vi "AlliGator Apply Calibration Phasor(s) v2.vi"(6 "Phasor Frequency":dbl[unit], 7 "Phasor Graph Ref":refnum<vi>, 8 "Error In":errorcluster, 9 "Plot Index (-1: last)":i32, 10 "Phasor Graph Ctrl Refnums":T1, 11 "AlliGator IV DVR":refnum<data-value>) -> (0 "Error Out":errorcluster, 1 "Apparent Phase Lifetime":dbl[unit], 2 "Calibrated Phasor":T2, 3 "AlliGator IV DVR":refnum<data-value>, 4 "Message":string)   [LabVIEW 2021, in "AlliGator Phasor Calibration.lvlib"]
doc: "Calibrates single, selected or all plots.\nUpdates the Phasor Graph and internal variables."
uses:
  AlliGator Phasor Calibration.lvlib
  Phasor/Phasor (g, s).ctl
  Internal Variables/AlliGator Internal Variables v2.ctl
  <vilib>/vision/Image Controls.llb/IMAQ Image.ctl
  Internal Variables/AlliGator Gate Image Set.ctl
  Files/AlliGator FLI Dataset Type.ctl
  Files/AlliGator Data Series Type.ctl
  Dual-Channel Datasets/AlliGator Dataset Channel.ctl
  Settings/AlliGator Gate Arithmetic.ctl
  Source Image/AlliGator Displayed Image.ctl
  Image/Named ROI Description.ctl
  Phasor Graph/AlliGator Decay Metadata v3.ctl
  Decay Analysis/Decay Preprocessing/AlliGator Decay Background Subtraction Info.ctl
  Decay Analysis/Decay Preprocessing/AlliGator Baseline Subtraction Method.ctl
  Graphs/XY Graph/XY Graph Plot Shift Parameters.ctl
  Graphs/XY Graph/XY Graph Plot Shift Method.ctl
  Decay Analysis/Decay Preprocessing/AlliGator Decay Extrapolation Parameters.ctl
  Phasor/Calibration Phasor (m, phi).ctl
  Phasor/Phasor Reference Series.ctl
  Phasor/Phasor Calibration Map v2.ctl
  Phasor Graph/AlliGator Raw Phasor Plot Data v5.ctl
  Phasor/Phasor Standard Deviation Options.ctl
  Phasor Plot/AlliGator Phasor Multi-Harmonic Data.ctl
  Phasor/Phasor Harmonic Data.ctl
  Decay Fit Parameter Map/AlliGator Decay Fit Options & Parameters v4.ctl
  Fits/IRF(X)PSED/Decay Fit Options v4.ctl
  Fits/Decay Convolution/Decay Model.ctl
  Fits/Residual Type.ctl
  Fits/IRF(X)PSED/Fit Weights Type v2.ctl
  Fits/Non-linear Fitting Method v2.ctl
  Fits/Fit Calculation Method.ctl
  Fits/Non-linear Fitting Algorithm.ctl
  Decay Analysis/Decay Fit/AlliGator Decay Fit Parameter Constraints 2.ctl
  Fits/IRF(X)PSED/Decay Fit Parameters In List.ctl
  Fits/IRF(X)PSED/MLE Baseline Offset Type.ctl
  Decay Analysis/Decay Preprocessing/AlliGator Decay Preprocessing Parameters.ctl
  Fits/IRF(X)PSED/Decay Fit Parameters & Derived Quantities List v2.ctl
  Fits/IRF(X)PSED/Decay Fit Result Constraint.ctl
  Decay Fit Parameter Map/AlliGator Parameter Maps Data.ctl
  GUI/AlliGator Phasor Graph Ctrl Refnums.ctl
  Phasor/Phasor Calibration Type.ctl
  Arrays/Arrays.lvlib
  Strings/Strings.lvlib
  Phasor/Phasor.lvlib
  Time/Time.lvlib
  Internal Variables/AlliGator Internal Variables.lvlib
  Image/Image.lvlib
  Files/AlliGator Files.lvlib
  Phasor Graph/AlliGator Phasor Graph.lvlib
  Decay Analysis/Decay Preprocessing/AlliGator Decay Preprocessing.lvlib
  Graphs/XY Graph/XY Graph Add-Ons.lvlib
  Phasor Plot/AlliGator Phasor Plot.lvlib
  Source Image/AlliGator Source Image.lvlib
  Fits/Fits.lvlib
  Decay Analysis/Decay Fit/AlliGator Decay Fit.lvlib
  GUI/AlliGator GUI.lvlib
  Settings/AlliGator Settings.lvlib
  Dual-Channel Datasets/AlliGator Dual-Channel Datasets.lvlib
  Decay Fit Parameter Map/AlliGator Decay Fit Parameter Map.lvlib
panel:
  out "# Plots":i32
  # "see the AlliGator License on the block diagram (Ctrl+E or Window:Show Block Diagram)"
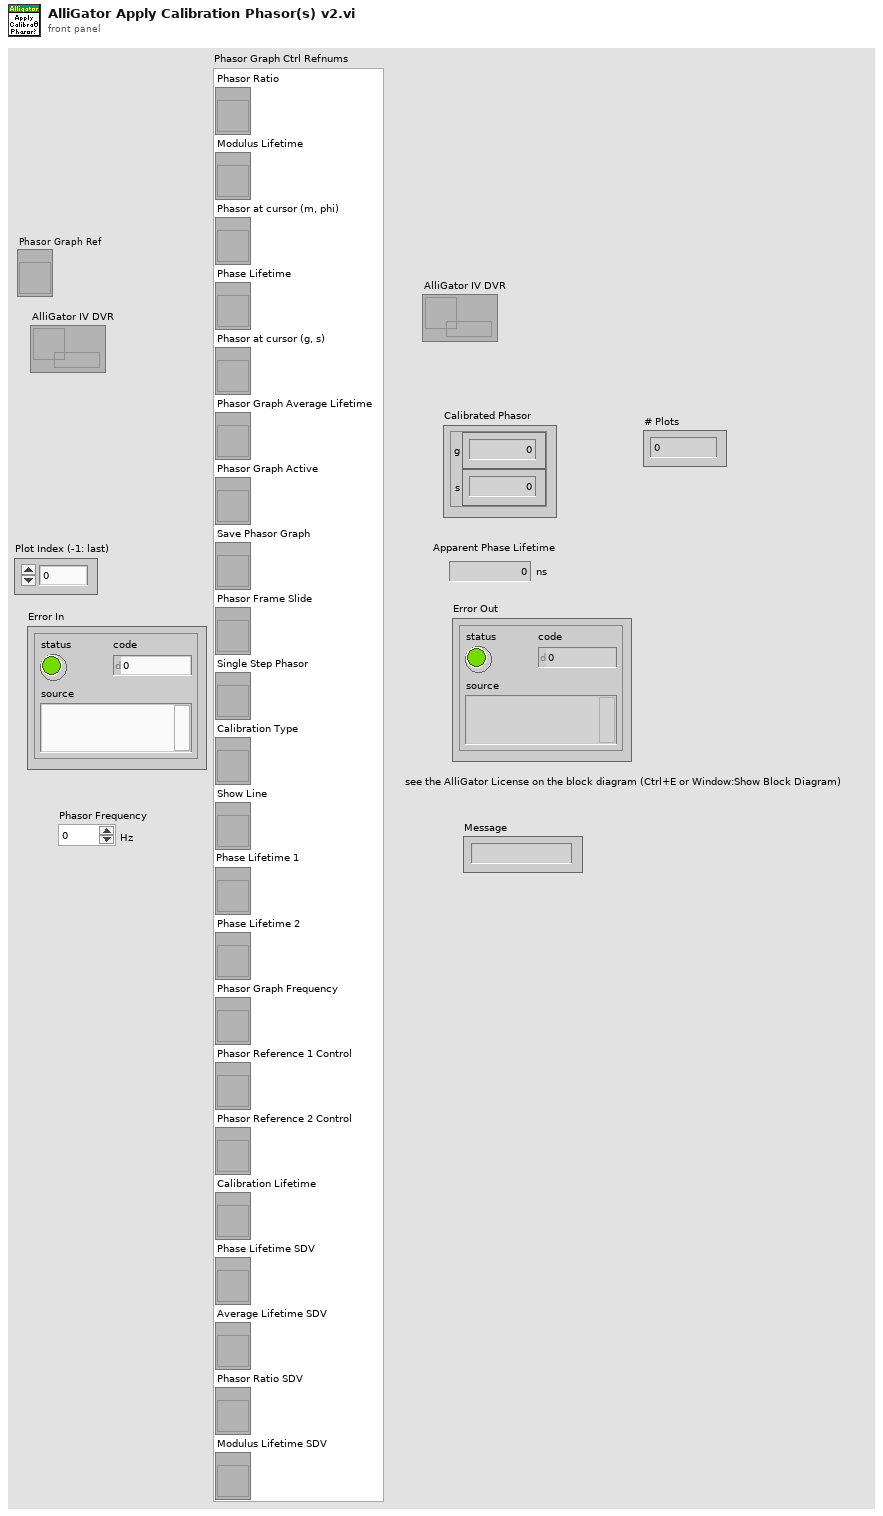
[diagram p1: front panel]
types:
  T1 = typedef "AlliGator GUI.lvlib/AlliGator Phasor Graph Ctrl Refnums.ctl" = cluster{"Phasor Ratio":refnum<vi>, "Modulus Lifetime":refnum<vi>, "Phasor at cursor (m, phi)":refnum<vi>, "Phase Lifetime":refnum<vi>, "Phasor at cursor (g, s)":refnum<vi>, "Phasor Graph Average Lifetime":refnum<vi>, "Phasor Graph Active":refnum<vi>, "Save Phasor Graph":refnum<vi>, "Phasor Frame Slide":refnum<vi>, "Single Step Phasor":refnum<vi>, "Calibration Type":refnum<vi>, "Show Line":refnum<vi>, "Phase Lifetime 1":refnum<vi>, "Phase Lifetime 2":refnum<vi>, "Phasor Graph Frequency":refnum<vi>, "Phasor Reference 1 Control":refnum<vi>, "Phasor Reference 2 Control":refnum<vi>, "Calibration Lifetime":refnum<vi>, "Phase Lifetime SDV":refnum<vi>, "Average Lifetime SDV":refnum<vi>, "Phasor Ratio SDV":refnum<vi>, "Modulus Lifetime SDV":refnum<vi>}
  T2 = typedef "Phasor.lvlib/Phasor (g, s).ctl" = cluster{"g":dbl, "s":dbl}
  T3 = typedef "AlliGator Internal Variables.lvlib/AlliGator Internal Variables v2.ctl" = cluster{"----------------------------- Images -----------------------------":u8, "Displayed Image":T4, "White Light Image":T4, "Mask Image":T4, "ROI Mask Image":T4, "Current Dataset Images 1":T5, "Background Dataset Images 1":T5, "Current Dataset Images 2":T5, "Background Dataset Images 2":T5, "Current Dataset Arithmetic Images":T5, "Accumulated Dataset Images 1":T5, "Accumulated Dataset Images 2":T5, "Accumulated Dataset Arithmetic Images":T5, "----------------------------- File Paths -----------------------------":u8, "Phasor Plot Image":T4, "Decay Fit Parameter Map Image":T4, "Parameter Map Image":T4, "Single Data Point Path":path, "White Light Image Path":path, "Mask Image Path":path, "Time-Series Folder":path, "[Time-Series Paths]":path[], "----------------------------- FLI Dataset -----------------------------":u8, "Current Dataset":i32, "Single Dataset Type":T6, "Current Folder":string, "AlliGator Data Series Type":T7, "# Datasets":i32, "Dual-Channel Dataset":bool, "Selected Channel Name":string, "Dataset Channel":T8, "Channel Arithmetic":T9, "Dual-Channel Background Dataset":bool, "Background Channel":T8, "Dual-Channel Accumulated Dataset":bool, "Start Time":dbl, "[Time-Series Timestamps]":dbl[], "[Intensity Corrections]":dbl[], "Time Series Script":bool, "Type of Displayed Image":T10, "Gate Image Slide":u16, "# Gates":i32, "ROIs":T11[], "----------------------------- Decays -----------------------------":u8, "ROI Decay":cluster{"t Array":dbl[], "I Array":dbl[]}, "Valid Decay":bool, "Decay  Metadata":T13, "Reference Decay Plot Name":string, "Reference Decay":cluster{"t Array":dbl[], "I Array":dbl[]}, "Decay Shift Plot":cluster{"Time Stamps":dbl[], "Decay Shifts":dbl[]}, "[Decays Max Values]":sgl[], "[Decays Min Values]":sgl[], "----------------------------- Calibration -----------------------------":u8, "Calibration Phasor":T19, "Calibration Phasor Series":T20, "Phasor Calibration Map":T21, "Calibration Map MD5 Digest":string, "----------------------------- Phasor Graph -----------------------------":u8, "Last Raw Phasor":T2, "Last Calibrated Phasor":T2, "Last Calibrated Phasor SDV":T2, "Phasor Graph:Phasor Plot":cluster{"g Array":dbl[], "s Array":dbl[]}, "Phasor Graph:Phasor SDV Plot":cluster{"g Array":dbl[], "s Array":dbl[]}, "[Phasor Graph:Raw Phasor Plots]":T22[], "Phasor Plot locked to Ref 1":i32, "[Phasor Plot(s) locked to Ref 1]":i32[], "[Phasor Plot(s) locked to Ref 2]":i32[], "[Pixel Phasors]":T2[], "----------------------------- Phasor Plot -----------------------------":u8, "[[Sum Image]]":dbl[][], "[[CSG Phasors]]":csg[][], "[[Valid Pixel?]]":bool[][], "[[Phasor Ratios]]":dbl[][], "[[Average Lifetimes]]":dbl[][], "Amplitude Weighted Average Lifetime":bool, "I/m/phi Dataset":cluster{"I/m/phi Dataset?":bool, "Base Frequency":dbl[unit], "Harmonic Orders":u8[]}, "Multi Phasor Plot Data":T24, "----------------------------- Decay Fit Parameter Map -----------------------------":u8, "Decay Fit Options & Parameters":T26, "Fit Options: Decay Preprocessing Parameters":T37, "Fit Options: Reference Decay":cluster{"t Array":dbl[], "I Array":dbl[]}, "Is Full Image Parameters Map":bool, "Is Single-Pixels Parameters Map":bool, "NLSF Parameters Map X Resolution":i32, "NLSF Parameters Map Y Resolution":i32, "[Single Decay Fit Parameters]":dbl[], "Fit Model":T28, "[[Multiple Decays Fit Parameters]]":dbl[][], "[[Multiple Decays Fit Parameter SDVs]]":dbl[][], "[[IRFs]]":dbl[][], "[ROI Descriptors]":T12[], "IRF Array Time Axis":dbl[], "Decay Array Time Axis":dbl[], "[Decay Fit Parameter Names]":T38[], "[Decay Sum]":dbl[], "Array of Decay Fit Result Constraints":T39[], "Selected ROIs Array":bool[], "----------------------------- Parameter Maps -----------------------------":u8, "[Map Set Names]":string[], "[Parameter Maps]":T40[], "[[User-defined Quantities]]":dbl[][], "User-defined Quantity":string}
  T4 = typedef "IMAQ Image.ctl" = refnum<image>
  T5 = typedef "AlliGator Internal Variables.lvlib/AlliGator Gate Image Set.ctl" = cluster{"SGL Image Max":T4, "SGL Image Sum":T4, "SGL Gate Images":T4[], "SGL Image Min":T4}
  T6 = typedef "AlliGator Files.lvlib/AlliGator FLI Dataset Type.ctl" = enum16{"HDF5 FLI Dataset", "Gate Image Folder", ".sdt FLI Dataset (Becker & Hickl)", ".ptu FLI Dataset (PicoQuant)", "SS1 FLI Dataset", "SS2 FLI Dataset", "I/m/phi Dataset", ".bin FLI Dataset (PicoQuant Binned)", ".bin FLI Dataset (Piccolo Binned)", ".mat FLI Dataset"}
  T7 = typedef "AlliGator Files.lvlib/AlliGator Data Series Type.ctl" = enum16{"Not a Supported Series", "Gate Images Folder Series", "SwissSPAD 2 Dataset Series", "B&H FLI Dataset Series", "PicoQuant PTU FLI Dataset Series", "PicoQuant BIN FLI Dataset Series", "Piccolo hist BIN FLI Dataset Series", "HDF5 FLI Dataset Series"}
  T8 = typedef "AlliGator Dual-Channel Datasets.lvlib/AlliGator Dataset Channel.ctl" = enum16{"G2", "INT"}
  T9 = typedef "AlliGator Settings.lvlib/AlliGator Gate Arithmetic.ctl" = enum16{"None", "INT-G2", "G2/INT*<INT>", "(1 - G2/INT)*<INT>"}
  T10 = typedef "AlliGator Source Image.lvlib/AlliGator Displayed Image.ctl" = enum16{"Single Gate", "Sum of All Gates", "Max of All Gates", "Min of All Gates", "-", "White Ligth Image", "Mask Image"}
  T11 = typedef "Image.lvlib/Named ROI Description.ctl" = cluster{"ROI Descriptor":T12, "ROI Name":string, "Overlay Color":u32}
  T12 = typedef "ROI Descriptor" = cluster{"Global Rectangle":i32[], "Contours":cluster{"ID":enum32{"External", "Internal"}, "Type":u32, "Coordinates":i32[]}[]}
  T13 = typedef "AlliGator Phasor Graph.lvlib/AlliGator Decay Metadata v3.ctl" = cluster{"ROI Descriptor":T12, "ROI Center":cluster{"X":i32, "Y":i32}, "Decay Background Subtraction Info":T14, "Decay Reverted":bool, "Decay Smoothened":bool, "Decay Straightened":bool, "Fitted Tau (Decay Straightening)":dbl, "Decay Shift Parameters":T16, "Decay Shifted":bool, "Decay Extrapolated":bool, "Decay Extrapolation Parameters":T18, "Decay Normalized":bool, "Fold Decay":bool, "# Folds":u32}
  T14 = typedef "AlliGator Decay Preprocessing.lvlib/AlliGator Decay Background Subtraction Info.ctl" = cluster{"Laser Period":dbl[unit], "Gate Duration":dbl[unit], "Baseline Subtraction Method":T15, "Background Definition Range":cluster{"Min Gate":dbl[unit], "Max Gate":dbl[unit]}, "Total Intensity w/o Bkgd Subtraction":dbl, "Bkgd-subtracted Intensity (exp)":dbl, "# Data Points":i32, "Background/Gate":dbl, "Fitted Lifetime":dbl[unit], "Bkgd-subtracted Intensity (theo)":dbl}
  T15 = typedef "AlliGator Decay Preprocessing.lvlib/AlliGator Baseline Subtraction Method.ctl" = enum16{"Mean", "Min", "Square Gated Single-Exponential", "File", "Constant"}
  T16 = typedef "XY Graph Add-Ons.lvlib/XY Graph Plot Shift Parameters.ctl" = cluster{"Type":T17, "Shift":dbl[unit], "Threshold":dbl, "Rotate":bool}
  T17 = typedef "XY Graph Add-Ons.lvlib/XY Graph Plot Shift Method.ctl" = enum16{"Default", "CFD", "Threshold", "Cross-Correlation"}
  T18 = typedef "AlliGator Decay Preprocessing.lvlib/AlliGator Decay Extrapolation Parameters.ctl" = cluster{"Additional Points":u32, "Head Fraction":dbl, "Fitted Tau":dbl, "Use Periodicity":bool, "Use Cursors":bool, "Tail Fraction":dbl}
  T19 = typedef "Phasor.lvlib/Calibration Phasor (m, phi).ctl" = cluster{"m":dbl, "phi":dbl, "Phasor Frequency":dbl[unit], "Reference Lifetime":dbl[unit]}
  T20 = typedef "Phasor.lvlib/Phasor Reference Series.ctl" = cluster{"m Array":dbl[], "phi Array":dbl[], "Phasor Frequency":dbl[unit], "Calibration Lifetime":dbl[unit]}
  T21 = typedef "Phasor.lvlib/Phasor Calibration Map v2.ctl" = cluster{"Phasor Frequency":dbl[unit], "Calibration Lifetime":dbl[unit], "ROI Centers":cluster{"X":i32, "Y":i32}[], "ROI Descriptors":T12[], "Map Resolution X":i32, "Map Resolution Y":i32, "z Array":cdb[]}
  T22 = typedef "AlliGator Phasor Graph.lvlib/AlliGator Raw Phasor Plot Data v5.ctl" = cluster{"Phasor Plot Name":string, "Raw Phasor Plot":T2[], "Phasor Frequency":dbl[unit], "[Decay Metadata]":T13[], "Raw Phasor Plot SDV":T2[], "Phasor SDV Options":T23, "[Calibration Phasor]":T19[], "Intensity Array":dbl[]}
  T23 = typedef "Phasor.lvlib/Phasor Standard Deviation Options.ctl" = cluster{"Compute Estimated SDV":bool, "# Replicas":u32, "Use Estimated Average Phasor":bool}
  T24 = typedef "AlliGator Phasor Plot.lvlib/AlliGator Phasor Multi-Harmonic Data.ctl" = cluster{"Base Frequency":dbl[unit], "# Harmonics":u8, "Harmonic Orders":u8[], "Phasor Plot Settings Checksum":u64, "Phasor Harmonic Data Array":T25[]}
  T25 = typedef "Phasor.lvlib/Phasor Harmonic Data.ctl" = cluster{"Phasor Harmonic Name":string, "Phasor Plot Settings Checksum":u64, "Phasor Frequency":dbl[unit], "Base Frequency":dbl[unit], "Harmonic Order":u8, "Phasor Plot Parameters":string, "Phasor Array [[CSG]]":csg[][], "Dataset File Path":path}
  T26 = typedef "AlliGator Decay Fit Parameter Map.lvlib/AlliGator Decay Fit Options & Parameters v4.ctl" = cluster{"SYNC Period":dbl[unit], "Fit Options":T27, "Fit Parameter Constraints":T34[], "MLE Baseline Offset":dbl, "MLE Baseline Offset Type":T36}
  T27 = typedef "Fits.lvlib/Decay Fit Options v4.ctl" = cluster{"Show Fit Residuals":bool, "Fit Model":T28, "Residual Type":T29, "Max Decay Percentile":dbl, "Min Decay Percentile":dbl, "Show Full Decay":bool, "Weights":T30, "Fitting Method":T31, "Compute Parameter Uncertainties":bool, "Periodic Boundaries":bool, "Model Calculation":T32, "Period":dbl[unit], "Termination Criteria":cluster{"Max Iterations":i32, "Max Function Calls":i32, "Max Time":dbl[unit], "Function Tolerance":dbl, "Parameter Tolerance":dbl, "Gradient Tolerance":dbl, "Min Lambda":dbl, "Max Lambda":dbl, "Initial Tick Count":u32}, "Offset Resolution":dbl[unit], "Use Local IRF":bool, "Fitting Algorithm":T33, "Show Confidence Interval ":bool, "Confidence Level":dbl}
  T28 = typedef "Fits.lvlib/Decay Model.ctl" = enum16{"1-Exponential", "2-Exponentials"}
  T29 = typedef "Fits.lvlib/Residual Type.ctl" = enum16{"Standard", "Normalized", "Reduced"}
  T30 = typedef "Fits.lvlib/Fit Weights Type v2.ctl" = enum16{"Unweighted", "1/Variance (Neyman)", "1/Variance (Pearson)", "Best of All"}
  T31 = typedef "Fits.lvlib/Non-linear Fitting Method v2.ctl" = enum16{"Least Square", "Least Absolute Residual", "Bisquare", "MLE", "-", "Best of All"}
  T32 = typedef "Fits.lvlib/Fit Calculation Method.ctl" = enum16{"Simulation", "Convolution", "Integration"}
  T33 = typedef "Fits.lvlib/Non-linear Fitting Algorithm.ctl" = enum16{"Levenberg-Marquardt", "Trust-Region Dogleg"}
  T34 = typedef "AlliGator Decay Fit.lvlib/AlliGator Decay Fit Parameter Constraints 2.ctl" = cluster{"Fit Parameter":T35, "Min Value":dbl, "Max Value":dbl, "Global":bool, "Used":bool}
  T35 = typedef "Fits.lvlib/Decay Fit Parameters In List.ctl" = enum16{"Offset", "Baseline", "A_1", "tau_1", "A_2", "tau_2"}
  T36 = typedef "Fits.lvlib/MLE Baseline Offset Type.ctl" = enum32{"Absolute", "Percentage"}
  T37 = typedef "AlliGator Decay Preprocessing.lvlib/AlliGator Decay Preprocessing Parameters.ctl" = cluster{"Background Subtraction":bool, "Straighten Decay":bool, "Reverse Gates":bool, "1-Normalized Decay":bool, "Smoothen Decay":bool, "Smoothing Parameter":dbl, "Shift Decay":bool, "Decay Shift Parameters":T16, "Extrapolate Decay":bool, "Additional Points":u32, "Head Fraction":dbl, "Pixel-Normalize Decay":bool, "Use Periodicity":bool, "Use Cursors":bool, "Tail Fraction":dbl, "Use Decay Pre-Processing":bool, "Fold Decay":bool, "# Folds":u32, "[0-1]-Normalized Decay":bool}
  T38 = typedef "Fits.lvlib/Decay Fit Parameters & Derived Quantities List v2.ctl" = enum16{"Offset", "Baseline", "A_1", "tau_1", "A_2", "tau_2", "<tau>_a", "f1_a", "f2_a", "<tau>_i", "f1_i", "f2_i", "-", "R^2", "Chi^2"}
  T39 = typedef "Fits.lvlib/Decay Fit Result Constraint.ctl" = cluster{"Fit Parameter":enum16{"Offset", "Baseline", "A_1", "tau_1", "A_2", "tau_2", "<tau>_a", "f1_a", "f2_a", "<tau>_i", "f1_i", "f2_i", "-", "R^2", "Chi^2", "Max Relative Residual", "<Residual ACF>", "Residual ACF SDV", "tau_2/tau_1"}, "Min Value":dbl, "Max Value":dbl, "Use Constraint":bool}
  T40 = typedef "AlliGator Decay Fit Parameter Map.lvlib/AlliGator Parameter Maps Data.ctl" = cluster{"Map Set Name":string, "[Parameter Names]":string[], "[[Parameters]]":dbl[][], "[[Parameter SDVs]]":dbl[][], "Decay Array Time Axis":dbl[], "[[IRFs]]":dbl[][], "IRF Array Time Axis":dbl[], "X Resolution":i32, "Y Resolution":i32, "Intensity Array":dbl[]}
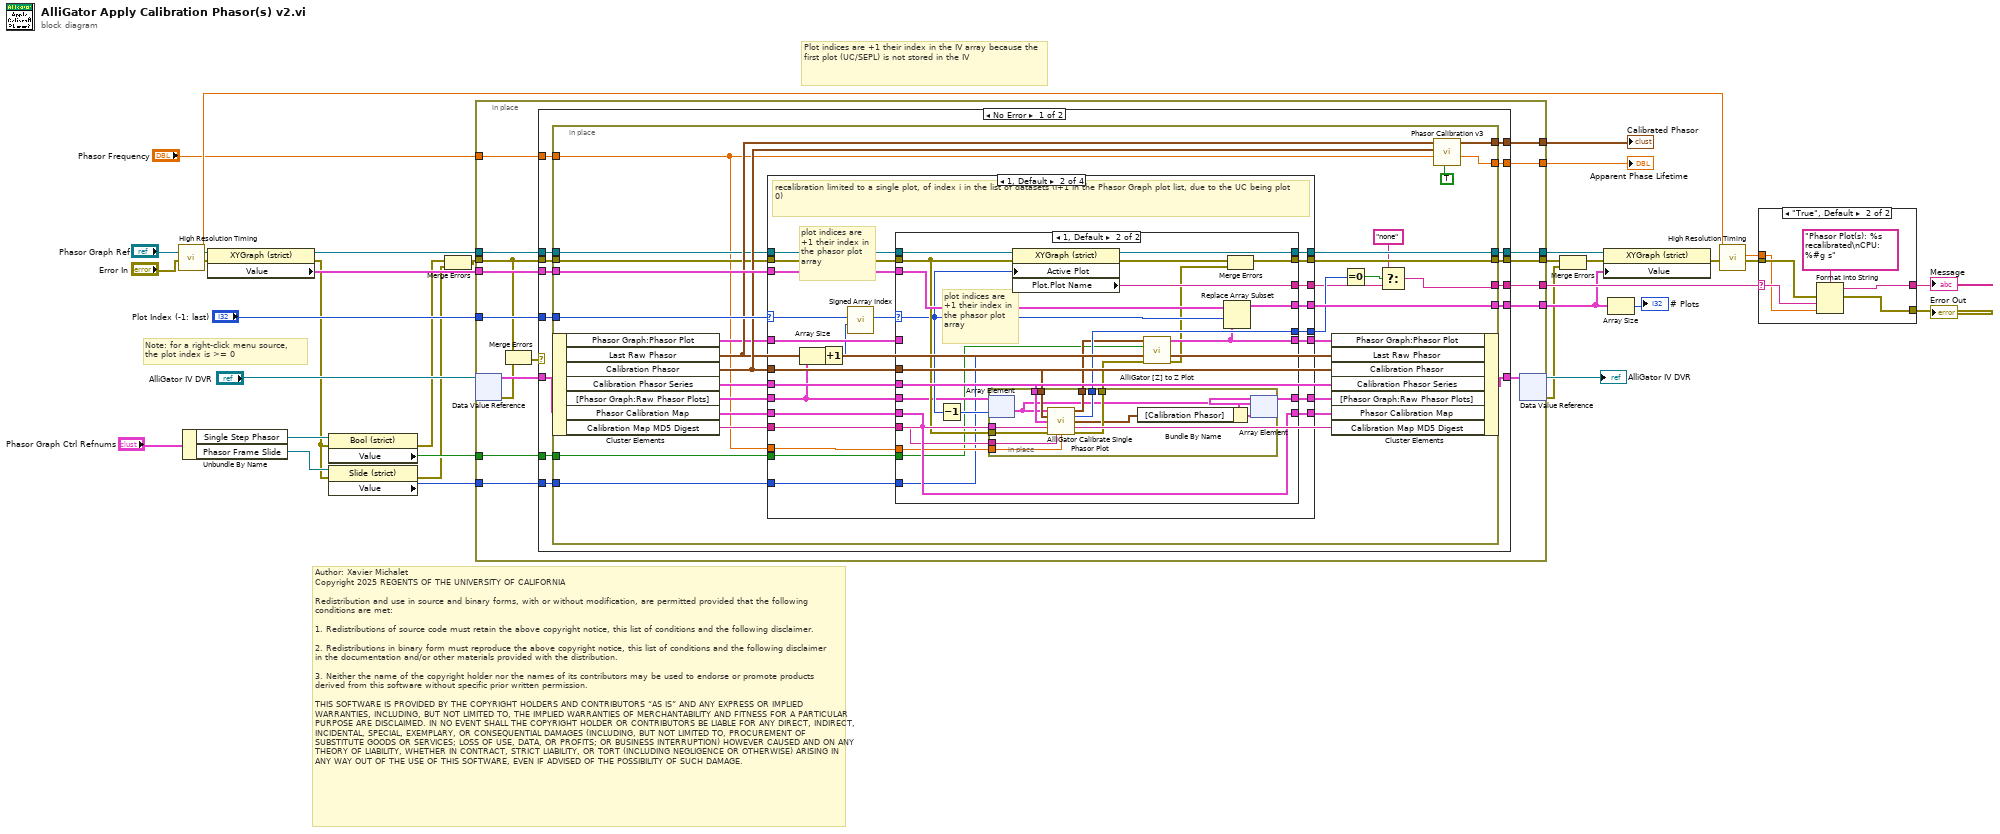
[diagram p0: block diagram]
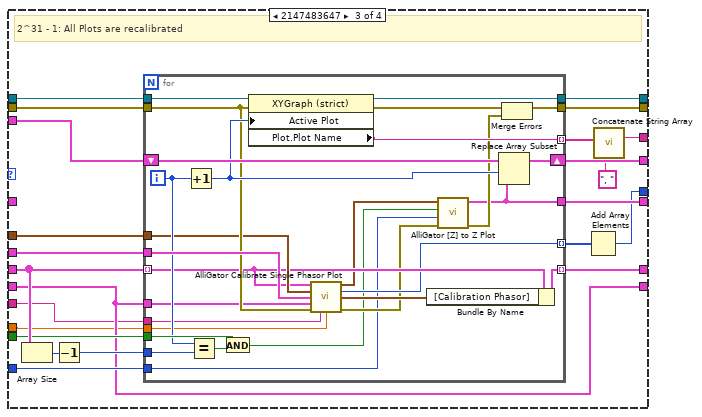
[diagram p4: hidden frame]
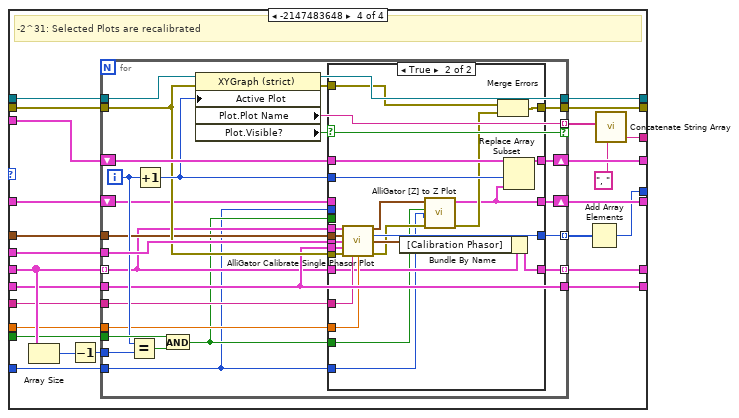
[diagram p5: hidden frame]
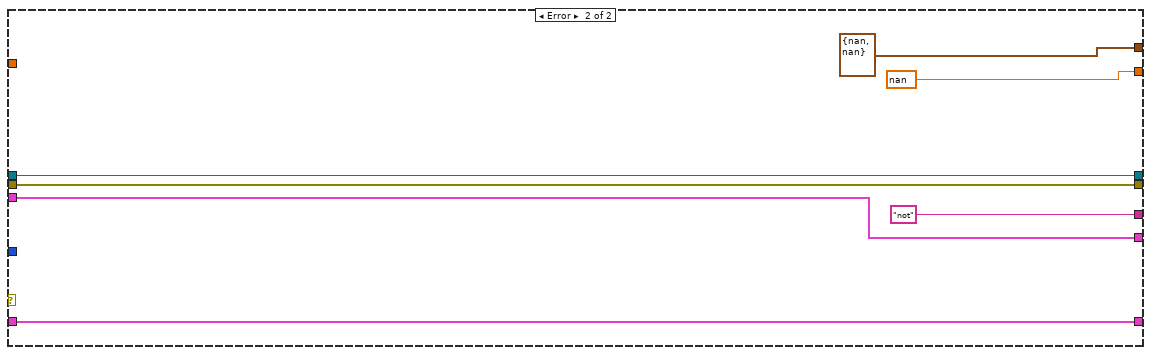
[diagram p7: hidden frame]
diagram:
  # "Author: Xavier Michalet\nCopyright 2025 REGENTS OF THE UNIVERSITY OF CALIFORNIA\n\nRedistribution and use in source and binary forms, with or without modification, are permitted provided that the following conditions are met:\n\n1. Redistributions of source code must retain the above copyright notice, this list of conditions and the following disclaimer.\n\n2. Redistributions in binary form must reproduce the above copyright notice, this list of conditions and the following disclaimer in the documentation and/or other materials provided with the distribution.\n\n3. Neither the name of the copyright holder nor the names of its contributors may be used to endorse or promote products derived from this software without specific prior written permission.\n\nTHIS SOFTWARE IS PROVIDED BY THE COPYRIGHT HOLDERS AND CONTRIBUTORS “AS IS” AND ANY EXPRESS OR IMPLIED WARRANTIES, INCLUDING, BUT NOT LIMITED TO, THE IMPLIED WARRANTIES OF MERCHANTABILITY AND FITNESS FOR A PARTICULAR PURPOSE ARE DISCLAIMED. IN NO EVENT SHALL THE COPYRIGHT HOLDER OR CONTRIBUTORS BE LIABLE FOR ANY DIRECT, INDIRECT, INCIDENTAL, SPECIAL, EXEMPLARY, OR CONSEQUENTIAL DAMAGES (INCLUDING, BUT NOT LIMITED TO, PROCUREMENT OF SUBSTITUTE GOODS OR SERVICES; LOSS OF USE, DATA, OR PROFITS; OR BUSINESS INTERRUPTION) HOWEVER CAUSED AND ON ANY THEORY OF LIABILITY, WHETHER IN CONTRACT, STRICT LIABILITY, OR TORT (INCLUDING NEGLIGENCE OR OTHERWISE) ARISING IN ANY WAY OUT OF THE USE OF THIS SOFTWARE, EVEN IF ADVISED OF THE POSSIBILITY OF SUCH DAMAGE."
  # "Note: for a right-click menu source,\nthe plot index is >= 0"
  # "Plot indices are +1 their index in the IV array because the first plot (UC/SEPL) is not stored in the IV"
  n1 = call "High Resolution Timing.vi"("Error In"="Error In") -> ("elapsed (relative) seconds"=w3:dbl, "Error Out"=w5:errorcluster)  [unwired: 16 in, 1 out]
  n2 = Unbundle By Name("Phasor Graph Ctrl Refnums") -> ("Single Step Phasor"=w15:refnum<vi>, "Phasor Frame Slide"=w13:refnum<vi>)
  n3 = property class="XYGraph (strict)"(reference="Phasor Graph Ref", error in=w5) -> (reference out=w25:refnum<vi>, error out=w11:errorcluster, "Value"=w28:cluster{"X Array":dbl[], "Y Array":dbl[]}[])
  n4 = property class="Bool (strict)"(reference=w15, error in=w11) -> (error out=w9:errorcluster, "Value"=w14:bool)  [unwired: 1 out]
  n5 = property class="Slide (strict)"(reference=w13, error in=w11) -> (error out=w8:errorcluster, "Value"=w12:i32)  [unwired: 1 out]
  n6 = Merge Errors(w9, w8) -> (w10:errorcluster)
  n7 = in-place {
    in-place-border: "Plot Index (-1: last)" -> [w48]
    in-place-border: w28 -> [w47]
    in-place-border: w12 -> [w46]
    in-place-border: [w45] -> w21
    in-place-border: [w44] -> w27
    in-place-border: [w43] -> w26
    in-place-border: w25 -> [w42]
    in-place-border: [w41] -> w23
    in-place-border: [w40] -> w24
    in-place-border: w10 -> [w37]
    in-place-border: [w39] -> w22
    in-place-border: w14 -> [w35]
    in-place-border: "Phasor Frequency" -> [w34]
    n8 = in-place-dvr #1("AlliGator IV DVR") -> (w50:T3, w38:errorcluster)
    n9 = Merge Errors(w37, w38) -> (w36:errorcluster)
    n10 = case shown="No Error" w36 {
      tunnel: w50 -> [w65 w300]
      tunnel: [w64 w300] -> w49
      tunnel: w48 -> [w63 _]
      tunnel: w47 -> [w62 w297]
      tunnel: w35 -> [w61 _]
      tunnel: w46 -> [w60 _]
      tunnel: [w59 w297] -> w45
      tunnel: [w58 T2 {"g"=nan, "s"=nan} ("Calibrated Phasor")] -> w44
      tunnel: [w57 dbl[unit] nan ("Calibrated Lifetime")] -> w43
      tunnel: w42 -> [w56 w298]
      tunnel: [w55 "not" ("Formatted String")] -> w41
      tunnel: [w54 w298] -> w40
      tunnel: [w53 w299] -> w39
      tunnel: w37 -> [w52 w299]
      tunnel: w34 -> [w51 _]
      frame No Error {
        n11 = in-place {
          in-place-border: w63 -> [w93]
          in-place-border: w62 -> [w92]
          in-place-border: w61 -> [w91]
          in-place-border: w60 -> [w90]
          in-place-border: [w89] -> w59
          in-place-border: [w85] -> w58
          in-place-border: [w77] -> w57
          in-place-border: w56 -> [w81]
          in-place-border: [w69] -> w55
          in-place-border: [w80] -> w54
          in-place-border: w52 -> [w79]
          in-place-border: [w78] -> w53
          in-place-border: w51 -> [w66]
          n12 = in-place-cluster #2(w65) -> ("Phasor Graph:Phasor Plot"=w82:cluster{"g Array":dbl[], "s Array":dbl[]}, "Last Raw Phasor"=w84:T2, "Calibration Phasor"=w86:T19, "Calibration Phasor Series"=w87:T20, "[Phasor Graph:Raw Phasor Plots]"=w88:T22[], "Phasor Calibration Map"=w75:T21, "Calibration Map MD5 Digest"=w73:string)
          n13 = case shown="1, Default" w93 {
            selector: w93 -> [_ w108 _ _]
            tunnel: w88 -> [w95 w121 w185 w238]
            tunnel: w92 -> [w97 w123 w188 w241]
            tunnel: w87 -> [_ w118 w187 w240]
            tunnel: w86 -> [_ w117 w186 w239]
            tunnel: w91 -> [_ w120 w182 w235]
            tunnel: w90 -> [_ w119 w181 w234]
            tunnel: [w97 w122 w180 w233] -> w89
            tunnel: [w96 w116 w179 w232] -> w83
            tunnel: w82 -> [w96 w115 _ w223]
            tunnel: w81 -> [w99 w114 w178 w231]
            tunnel: [_ w112 w175 w228] -> w70
            tunnel: [w99 w113 w177 w230] -> w80
            tunnel: w79 -> [w98 w111 w173 w226]
            tunnel: [w98 w110 w172 w225] -> w78
            tunnel: w75 -> [w94 w109 w170 w224]
            tunnel: [w95 w103 w171 w222] -> w76
            tunnel: [w94 w104 w170 w221] -> w74
            tunnel: w73 -> [_ w102 w169 w220]
            tunnel: [_ w101 w167 w218] -> w72
            tunnel: w66 -> [_ w100 w166 w217]
            frame 0 {
              # "UC: do nothing"
            }
            frame 1, Default {
              # "plot indices are\n+1 their index in the phasor plot array"
              # "recalibration limited to a single plot, of index i in the list of datasets (i+1 in the Phasor Graph plot list, due to the UC being plot 0)"
              n14 = Array Size(array=w121) -> (size(s)=w107:i32)
              n15 = Increment(x=w107) -> (x+1=w105:i32)
              n16 = call "Signed Array Index.vi"("Array Size"=w105, "Array Index in"=w108) -> ("Array Index out"=w106:i32)  [unwired: 9 in]
              n17 = case shown="1, Default" w106 {
                selector: w106 -> [_ w143]
                tunnel: w123 -> [w127 w153]
                tunnel: [w127 w152] -> w122
                tunnel: w121 -> [w124 w138]
                tunnel: w120 -> [_ w132]
                tunnel: w119 -> [_ w131]
                tunnel: w118 -> [_ w151]
                tunnel: [w126 w133] -> w116
                tunnel: w114 -> [w129 w150]
                tunnel: [_ w149] -> w112
                tunnel: [w129 w148] -> w113
                tunnel: w111 -> [w128 w146]
                tunnel: [w128 w145] -> w110
                tunnel: w117 -> [_ w144]
                tunnel: w109 -> [w125 w142]
                tunnel: w115 -> [w126 _]
                tunnel: [w125 w142] -> w104
                tunnel: [w124 w137] -> w103
                tunnel: w102 -> [_ w141]
                tunnel: [_ w140] -> w101
                tunnel: w100 -> [_ w139]
                frame 0 {
                  # "UC: do nothing"
                }
                frame 1, Default {
                  # "plot indices are\n+1 their index in the phasor plot array"
                  n18 = Decrement(x=w143) -> (x-1=w136:i32)
                  n19 = in-place {
                    in-place-border: w151 -> [w165]
                    in-place-border: [w164] -> w135
                    in-place-border: w146 -> [w163]
                    in-place-border: [w162] -> w134
                    in-place-border: w144 -> [w161]
                    in-place-border: w142 -> [w160]
                    in-place-border: w141 -> [w159]
                    in-place-border: [w158] -> w140
                    in-place-border: w139 -> [w157]
                    n20 = in-place-array #3(w138, w136) -> (w156:T22)
                    n21 = call "AlliGator Calibrate Single Phasor Plot.vi"("Raw Phasor Plot"=w156, "Calibration Phasor"=w161, "Calibration Phasor Series"=w165, "Phasor Calibration Map"=w160, "Error In"=w163, "Calibration Map MD5 Digest"=w159, "Phasor Frequency"=w157) -> ("[Calibrated Phasor]"=w164:T2[], "# Recalibrated Phasors"=w158:i32, "[Calibration Phasor]"=w155:T19[], "Error Out"=w162:errorcluster)  [unwired: 5 in]
                    n22 = Bundle By Name(cluster=w156, "[Calibration Phasor]"=w155) -> (w154:T22)
                    n23 = in-place-array #3(w154) -> (w137:T22[])  [unwired: 1 out]
                  }
                  n24 = property class="XYGraph (strict)"(reference=w150, error in=w146, "Active Plot"=w143) -> (reference out=w148:refnum<vi>, error out=w147:errorcluster, "Plot.Plot Name"=w149:string)
                  n25 = call "AlliGator [Z] to Z Plot.vi"("Error In"=w134, "Phasor Graph Slide (-1: last)"=w131, "Single Point Display? (F)"=w132, "[Calibrated Phasor]"=w135) -> ("Error Out"=w130:errorcluster, "Calibrated Phasor Plot"=w133:cluster{"Array":dbl[], "Array":dbl[]})  [unwired: 6 in]
                  n26 = Replace Array Subset(array=w153, new element=w133, index=w143) -> (w152:cluster{"X Array":dbl[], "Y Array":dbl[]}[])
                  n27 = Merge Errors(w147, w130) -> (w145:errorcluster)
                }
              }
            }
            frame 2147483647 {
              # "2^31 - 1: All Plots are recalibrated"
              n28 = Array Size(array=w185) -> (size(s)=w184:i32)
              n29 = Decrement(x=w184) -> (x-1=w183:i32)
              n30 = for {
                shift-right: [w215] -> w180
                shift-left: w188 -> [w216]
                tunnel: w187 -> [w214]
                tunnel: w186 -> [w202]
                tunnel: w183 -> [w213]
                tunnel: w182 -> [w212]
                tunnel: w181 -> [w189]
                tunnel: w185 -> [w200] mode=indexing
                tunnel: [w190] -> w179
                tunnel: w178 -> [w210]
                tunnel: [w209] -> w177
                tunnel: [w208] -> w176 mode=indexing
                tunnel: w173 -> [w204]
                tunnel: [w203] -> w172
                tunnel: w170 -> [w201]
                tunnel: [w197] -> w171 mode=indexing
                tunnel: w169 -> [w199]
                tunnel: [w195] -> w168 mode=indexing
                tunnel: w166 -> [w198]
                i -> [w206]
                n31 = Increment(x=w206) -> (x+1=w205:i32)
                n32 = Equal?(x=w206, y=w213) -> (x = y?=w211:bool)
                n33 = And(x=w212, y=w211) -> (x .and. y?=w191:bool)
                n34 = property class="XYGraph (strict)"(reference=w210, error in=w204, "Active Plot"=w205) -> (reference out=w209:refnum<vi>, error out=w207:errorcluster, "Plot.Plot Name"=w208:string)
                n35 = call "AlliGator Calibrate Single Phasor Plot.vi"("Raw Phasor Plot"=w200, "Calibration Phasor"=w202, "Calibration Phasor Series"=w214, "Phasor Calibration Map"=w201, "Error In"=w204, "Calibration Map MD5 Digest"=w199, "Phasor Frequency"=w198) -> ("[Calibrated Phasor]"=w194:T2[], "# Recalibrated Phasors"=w195:i32, "[Calibration Phasor]"=w196:T19[], "Error Out"=w193:errorcluster)  [unwired: 5 in]
                n36 = Bundle By Name(cluster=w200, "[Calibration Phasor]"=w196) -> (w197:T22)
                n37 = call "AlliGator [Z] to Z Plot.vi"("Error In"=w193, "Phasor Graph Slide (-1: last)"=w189, "Single Point Display? (F)"=w191, "[Calibrated Phasor]"=w194) -> ("Error Out"=w192:errorcluster, "Calibrated Phasor Plot"=w190:cluster{"Array":dbl[], "Array":dbl[]})  [unwired: 6 in]
                n38 = Replace Array Subset(array=w216, new element=w190, index=w205) -> (w215:cluster{"X Array":dbl[], "Y Array":dbl[]}[])
                n39 = Merge Errors(w207, w192) -> (w203:errorcluster)
              }
              n40 = Add Array Elements(numeric array=w168) -> (sum=w167:i32)
              n41 = call "Concatenate String Array.vi"("Separator (TAB)"=", ", "String Array"=w176) -> ("Formatted String"=w175:string)  [unwired: 9 in]
            }
            frame -2147483648 {
              # "-2^31: Selected Plots are recalibrated"
              n42 = Array Size(array=w238) -> (size(s)=w237:i32)
              n43 = Decrement(x=w237) -> (x-1=w236:i32)
              n44 = for {
                shift-right: [w266] -> w233
                shift-left: w241 -> [w267]
                tunnel: w240 -> [w265]
                tunnel: w239 -> [w253]
                tunnel: w236 -> [w264]
                tunnel: w235 -> [w263]
                tunnel: w234 -> [w242]
                tunnel: w238 -> [w245] mode=indexing
                tunnel: w231 -> [w260]
                tunnel: [w259] -> w230
                tunnel: [w252] -> w229 mode=indexing if=w251
                tunnel: w226 -> [w255]
                tunnel: [w254] -> w225
                tunnel: w224 -> [w249]
                shift-right: [w261] -> w232
                shift-left: w223 -> [w250]
                tunnel: [w244] -> w222 mode=indexing
                tunnel: [w249] -> w221
                tunnel: w220 -> [w248]
                tunnel: [w247] -> w219 mode=indexing
                tunnel: w217 -> [w246]
                i -> [w257]
                n45 = Equal?(x=w257, y=w264) -> (x = y?=w262:bool)
                n46 = Increment(x=w257) -> (x+1=w256:i32)
                n47 = And(x=w263, y=w262) -> (x .and. y?=w243:bool)
                n48 = property class="XYGraph (strict)"(reference=w260, error in=w255, "Active Plot"=w256) -> (reference out=w259:refnum<vi>, error out=w258:errorcluster, "Plot.Plot Name"=w252:string, "Plot.Visible?"=w251:bool)
                n49 = case shown="True" w251 {
                  tunnel: w267 -> [w270 w293]
                  tunnel: [w270 w292] -> w266
                  tunnel: w265 -> [_ w291]
                  tunnel: [w269 w272] -> w261
                  tunnel: w258 -> [w271 w290]
                  tunnel: w256 -> [_ w289]
                  tunnel: w255 -> [_ w288]
                  tunnel: [w271 w287] -> w254
                  tunnel: w253 -> [_ w286]
                  tunnel: w245 -> [_ w285]
                  tunnel: w249 -> [_ w284]
                  tunnel: w250 -> [w269 _]
                  tunnel: w243 -> [_ _]
                  tunnel: w242 -> [_ _]
                  tunnel: w248 -> [_ w283]
                  tunnel: [_ w282] -> w247
                  tunnel: w246 -> [_ w281]
                  tunnel: w245 -> [w268 w280]
                  tunnel: [w268 w279] -> w244
                  tunnel: w243 -> [_ w275]
                  tunnel: w242 -> [_ w274]
                  frame False {
                  }
                  frame True {
                    n50 = call "AlliGator Calibrate Single Phasor Plot.vi"("Raw Phasor Plot"=w285, "Calibration Phasor"=w286, "Calibration Phasor Series"=w291, "Phasor Calibration Map"=w284, "Error In"=w288, "Calibration Map MD5 Digest"=w283, "Phasor Frequency"=w281) -> ("[Calibrated Phasor]"=w277:T2[], "# Recalibrated Phasors"=w282:i32, "[Calibration Phasor]"=w278:T19[], "Error Out"=w276:errorcluster)  [unwired: 5 in]
                    n51 = Bundle By Name(cluster=w280, "[Calibration Phasor]"=w278) -> (w279:T22)
                    n52 = call "AlliGator [Z] to Z Plot.vi"("Error In"=w276, "Phasor Graph Slide (-1: last)"=w274, "Single Point Display? (F)"=w275, "[Calibrated Phasor]"=w277) -> ("Error Out"=w273:errorcluster, "Calibrated Phasor Plot"=w272:cluster{"Array":dbl[], "Array":dbl[]})  [unwired: 6 in]
                    n53 = Merge Errors(w290, w273) -> (w287:errorcluster)
                    n54 = Replace Array Subset(array=w293, new element=w272, index=w289) -> (w292:cluster{"X Array":dbl[], "Y Array":dbl[]}[])
                  }
                }
              }
              n55 = Add Array Elements(numeric array=w219) -> (sum=w218:i32)
              n56 = call "Concatenate String Array.vi"("Separator (TAB)"=", ", "String Array"=w229) -> ("Formatted String"=w228:string)  [unwired: 9 in]
            }
          }
          n57 = in-place-cluster #2("Phasor Graph:Phasor Plot"=w83, "Last Raw Phasor"=w84, "Calibration Phasor"=w86, "Calibration Phasor Series"=w87, "[Phasor Graph:Raw Phasor Plots]"=w76, "Phasor Calibration Map"=w74, "Calibration Map MD5 Digest"=w73) -> (w64:T3)
          n58 = Equal To 0?(x=w72) -> (x = 0?=w71:bool)
          n59 = Select(t="none", s=w71, f=w70) -> (s? t:f=w69:string)
          n60 = call "Phasor Calibration v3.vi"("Compute Lifetimes? (F)"=TRUE ("Init?"), "Phasor Frequency"=w66, "Calibration Phasor"=w86, "Measured Phasor"=w84) -> ("Calibrated Phase Lifetime"=w77:dbl[unit], "Calibrated Phasor"=w85:T2)  [unwired: 2 in, 4 out]
        }
      }
      frame Error {
      }
    }
    n61 = in-place-dvr #1(w49) -> (→"AlliGator IV DVR":refnum<data-value>, w17:errorcluster)
  }
  "Calibrated Phasor" <- w27
  "Apparent Phase Lifetime" <- w26
  n62 = Merge Errors(w22, w17) -> (w18:errorcluster)
  n63 = property class="XYGraph (strict)"(reference=w24, error in=w18, "Value"=w21) -> (error out=w19:errorcluster)  [unwired: 1 out]
  n64 = Array Size(array=w21) -> (size(s)=→"# Plots":i32)
  n65 = call "High Resolution Timing.vi"("relative seconds (NaN)"=w3, "Error In"=w19) -> ("elapsed (relative) seconds"=w2:dbl, "Error Out"=w4:errorcluster)  [unwired: 15 in, 1 out]
  n66 = case shown="\"True\", Default" w23 {
    selector: w23 -> [w302 w306]
    tunnel: [w302 w307] -> w7
    tunnel: w4 -> [w301 w305]
    tunnel: [w301 w304] -> w6
    tunnel: w2 -> [_ w303]
    frame "" {
    }
    frame "True", Default {
      n67 = Format Into String(format string="Phasor Plot(s): %s recalibrated\nCPU: %#g s", error in=w305, w306, w303) -> (resulting string=w307:string, error out=w304:errorcluster)  [unwired: 1 in]
    }
  }
  "Error Out" <- w6
  "Message" <- w7
